vi "ProcessSensorData.vi"(8 "error in (no error)":errorcluster, 10 "clSensorData":T1, 11 "Class In":refnum<class "PmuAnalysis.lvclass">) -> (0 "error out":errorcluster, 3 "Class Out":refnum<class "PmuAnalysis.lvclass">)   [LabVIEW 2014, in "AnalysisPlugins.lvlib" / "PmuAnalysis.lvclass"]
uses:
  PmuAnalysis.lvclass
  AnalysisPluginBaseClass/Typedefs/clSensorData.ctl
  Typedefs/PmuData.ctl
  AnalysisPluginBaseClass/AnalysisPluginsBase.lvclass/AnalysisPluginsBase.ctl
  PmuAnalysis.lvclass/PmuAnalysis.ctl
  AnalysisPluginBaseClass/Accessors/Write AnalysisTime.vi
  Accessors/Write PmuReport.vi
  <vilib>/Utility/error.llb/Error Cluster From Error Code.vi
  <vilib>/ErrorRing/Error Ring.xnode
  AnalysisPluginBaseClass/AnalysisPluginsBase.lvclass
panel:
  out "Waveform Chart":dbl(graph)
  out "time stamp":timestamp format="%^<%.3X\n%x>T"
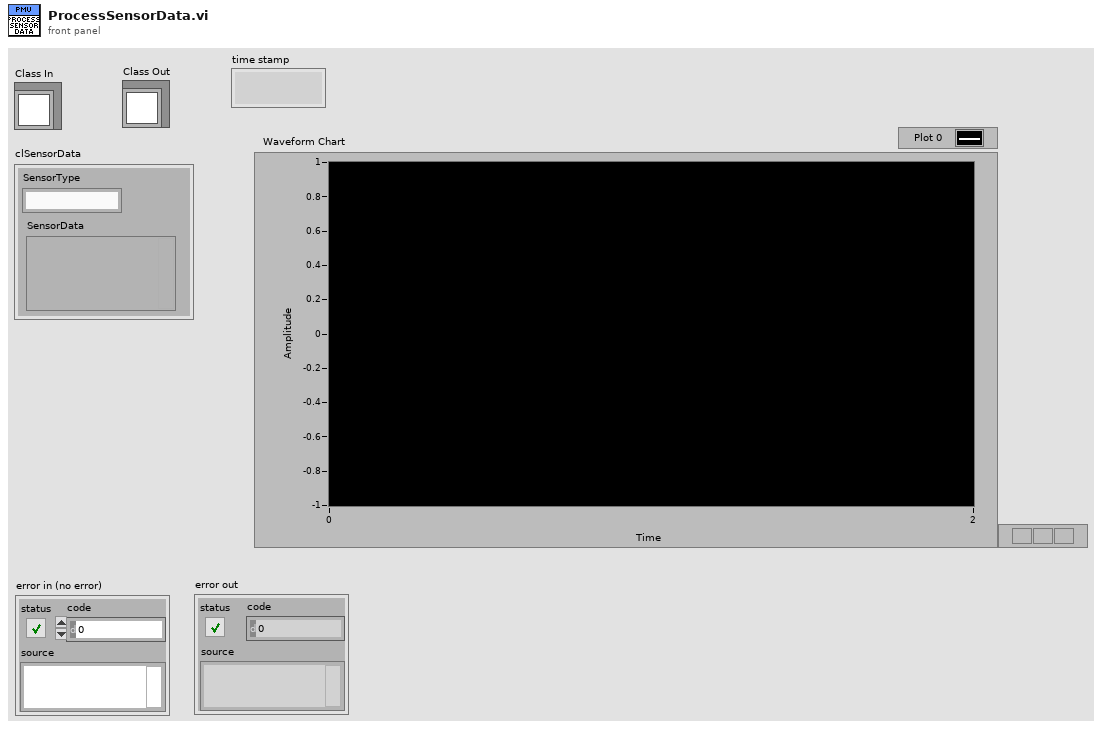
[diagram p1: front panel]
types:
  T1 = typedef "AnalysisPlugins.lvlib/AnalysisPluginsBase.lvclass/clSensorData.ctl" = cluster{"SensorType":string, "SensorData":variant}
  T2 = typedef "AnalysisPlugins.lvlib/PmuAnalysis.lvclass/PmuData.ctl" = cluster{"Timestamp":dbl, "Synx":cdb[], "Freq":dbl, "ROCOF":dbl, "ID":i16}
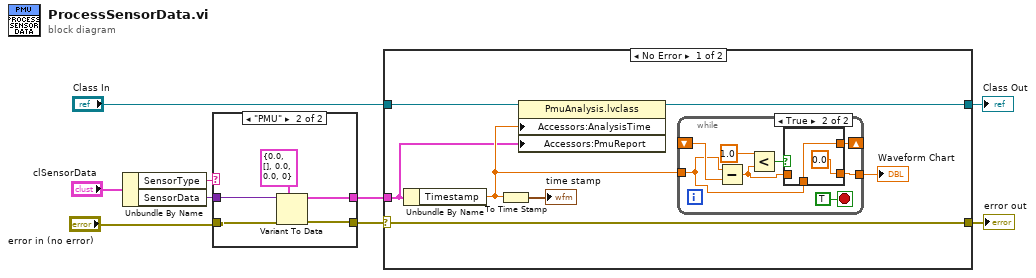
[diagram p0: block diagram]
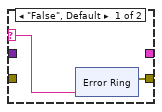
[diagram p4: hidden frame]
diagram:
  n1 = Unbundle By Name("clSensorData") -> ("SensorType"=w7:string, "SensorData"=w6:variant)
  n2 = case shown="\"PMU\"" w7 {
    selector: w7 -> [w10 _]
    tunnel: [w11 w20] -> w2
    tunnel: w6 -> [_ w23]
    tunnel: "error in (no error)" -> [_ w22]
    tunnel: [_ w19] -> w3
    frame "False", Default {
      n3 = xnode "Error Ring"("parameter 0"=w10) -> ("error out"=w11:errorcluster)
    }
    frame "PMU" {
      n4 = Variant To Data(error in=w22, type=T2 {"Timestamp"=0.0, "Synx"=[], "Freq"=0.0, "ROCOF"=0.0, "ID"=0} ("PmuReport"), Variant=w23) -> (data=w19:T2, error out=w20:errorcluster)
    }
  }
  n5 = case shown="No Error" w2 {
    selector: w2 -> [w24 w43]
    tunnel: "Class In" -> [w30 w44]
    tunnel: [w28 w44] -> w4
    tunnel: w3 -> [w25 _]
    tunnel: [w24 w43] -> w1
    frame No Error {
      n6 = Unbundle By Name(w25) -> ("Timestamp"=w27:dbl)
      n7 = To Time Stamp(1:w27) -> (0:→"time stamp":timestamp)
      n8 = property class="PmuAnalysis.lvclass"(reference=w30, "Accessors:AnalysisTime"=w27, "Accessors:PmuReport"=w25) -> (reference out=w28:refnum<class "PmuAnalysis.lvclass">)  [unwired: 1 in, 1 out]
      n9 = while {
        tunnel: w27 -> [w32]
        shift-right: [w31] -> _
        shift-left: _ -> [w34]
        tunnel: [w33] -> w26
        stop <- TRUE stop-if-true
        n10 = Subtract(x=w32, y=w34) -> (x-y=w35:dbl)
        n11 = Less?(x=1.0, y=w35) -> (x < y?=w36:bool)
        n12 = case shown="True" w36 {
          tunnel: w35 -> [w40 _]
          tunnel: [w40 0.0] -> w33
          tunnel: w32 -> [w39 w41]
          tunnel: [w39 w41] -> w31
          frame False {
          }
          frame True {
          }
        }
      }
      "Waveform Chart" <- w26
    }
    frame Error {
    }
  }
  "Class Out" <- w4
  "error out" <- w1
